vi "sweep_settings_to_command.vi"(11 "sweep_param":dbl[](array[numeric])) -> (3 "scan_command":string)   [LabVIEW 2025]
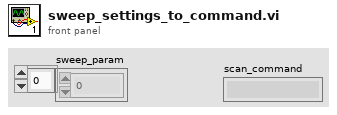
[diagram p1: front panel]
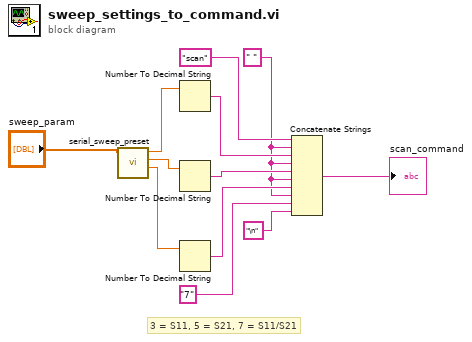
[diagram p0: block diagram]
diagram:
  w7 = " "
  # "3 = S11, 5 = S21, 7 = S11/S21"
  n1 = call "serial_sweep_preset.vi"("sweep_data"="sweep_param") -> ("sweep_points"=w2:dbl, "sweep_stop"=w3:dbl, "sweep_start"=w4:dbl)  [unwired: 8 in]
  n2 = Number To Decimal String(number=w4) -> (decimal integer string=w11:string)  [unwired: 1 in]
  n3 = Number To Decimal String(number=w3) -> (decimal integer string=w10:string)  [unwired: 1 in]
  n4 = Number To Decimal String(number=w2) -> (decimal integer string=w9:string)  [unwired: 1 in]
  n5 = Concatenate Strings("scan", w7, w11, w7, w10, w7, w9, w7, "7", "\n") -> (→"scan_command":string)
